vi "M227 Test Panel.vi"() -> ()   [LabVIEW 2020]
uses:
  <vilib>/Instr/_visa.llb/VISA Configure Serial Port (Instr).vi
panel:
  out "Waiting for Reply":bool
  out "Axis 3 Position":dbl
  out "Axis 2 Position":dbl
  out "Axis 1 Position":dbl
  in  "Move All (mm)":dbl
  out "Last Error":errorcluster
  out "Command History":string
  out "Reply":string
  in  "Command":string
  out "Connected":bool
  in  "Quit":bool
  in  "COM Port":refnum<visa-resource-name>="COM4"
  # "Example Commands:\n\nGet info for contoller 1\n1 *IDN?\n\nGet info for contoller 2\n2 *IDN?\n\nGet info for contoller 3\n3 *IDN?\n\nGet position of axis 1\n1 POS?\n\nGet position of axis 2\n2 POS?\n\nGet position of axis 2\n3 POS?\n\nMove axis 1 to a position of +1.5 mm\n1 MOV 1 1.5\n\nMove axis 2 to a position of +1.5 mm\n2 MOV 1 1.5\n\nMove axis 2 to a position of +1.5 mm\n3 MOV 1 1.5"
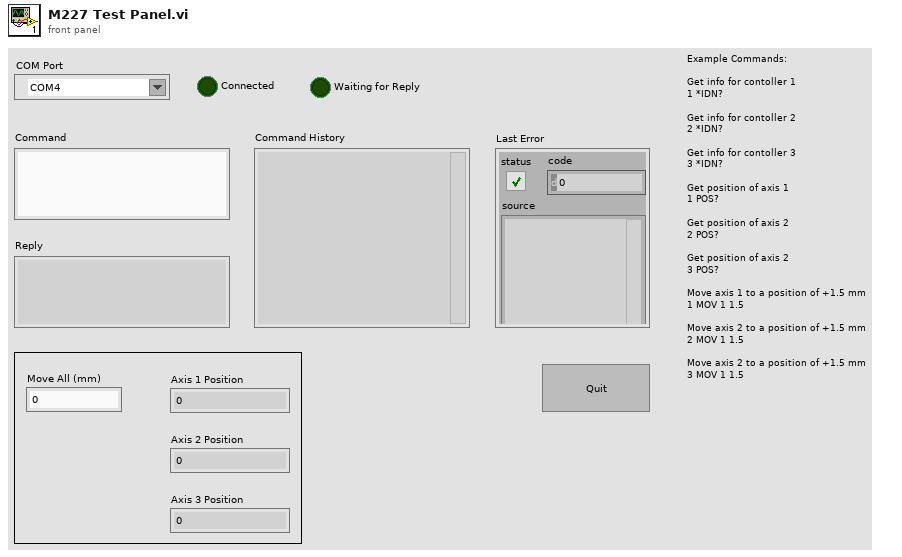
[diagram p1: front panel]
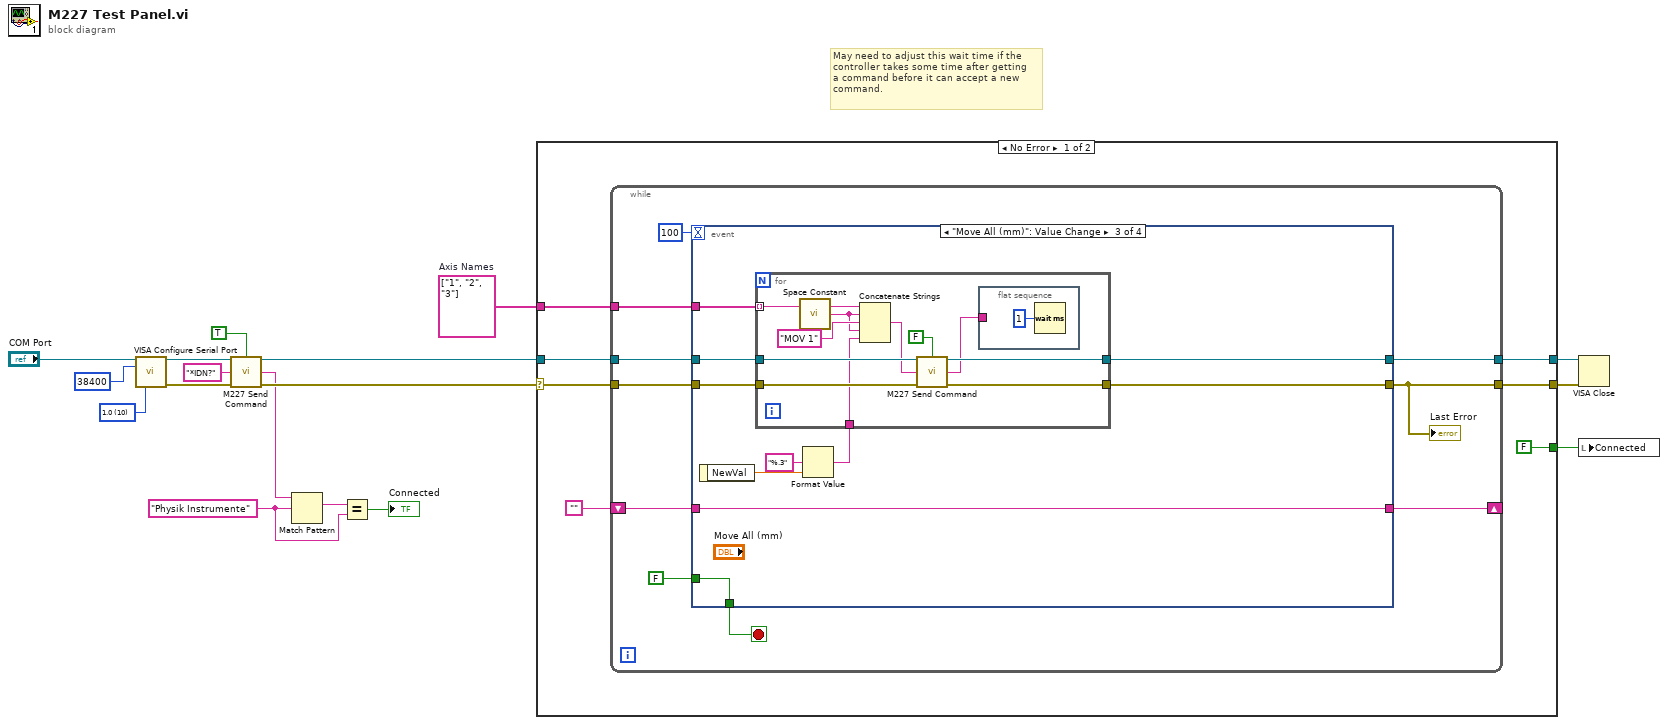
[diagram p0: block diagram]
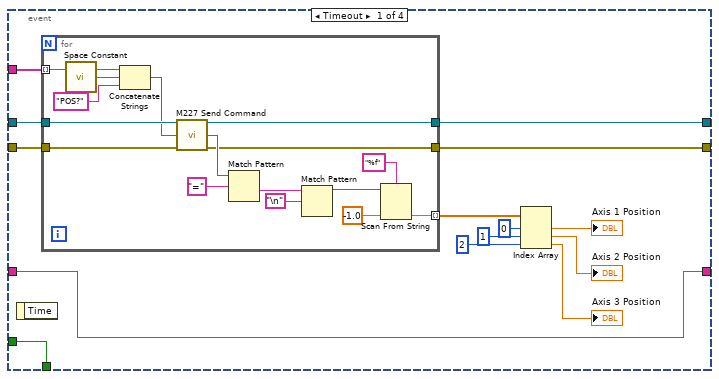
[diagram p2: hidden frame]
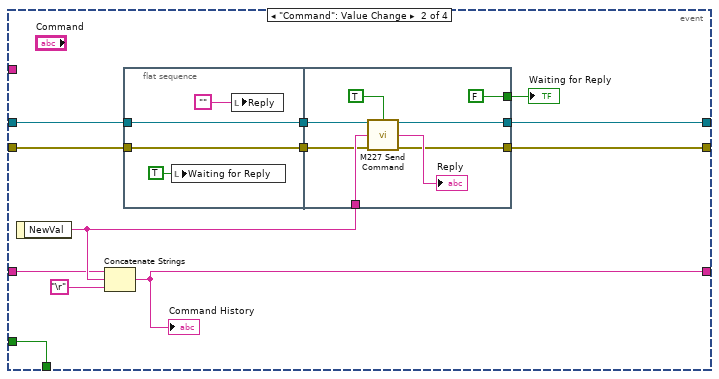
[diagram p3: hidden frame]
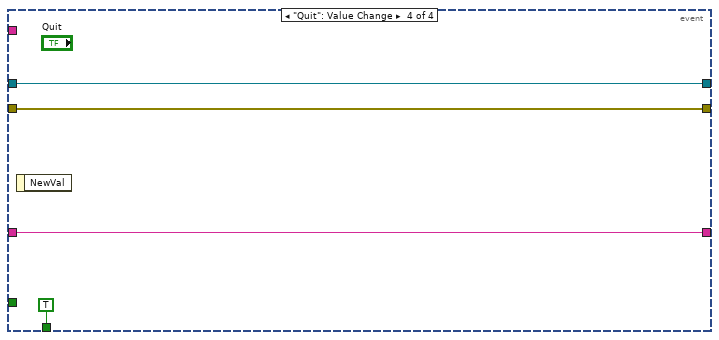
[diagram p4: hidden frame]
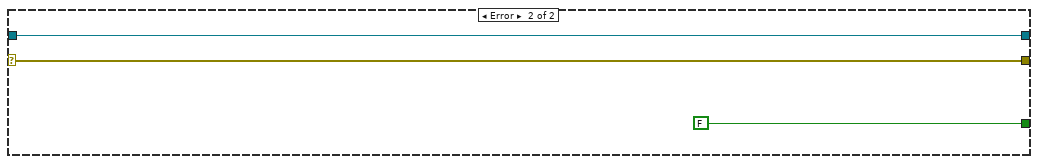
[diagram p5: hidden frame]
diagram:
  w1 = string[] ["1", "2", "3"]  # Axis Names
  w4 = "Physik Instrumente" ("regular expression")
  w17 = u16 10 items=["1.0"=10, "1.5"=15, "2.0"=20] ("stop bits (10: 1 bit)")
  # "May need to adjust this wait time if the\ncontroller takes some time after getting\na command before it can accept a new\ncommand."
  n1 = call-poly "VISA Configure Serial Port"("VISA resource name"="COM Port", "baud rate (9600)"=u32 38400, "stop bits (10: 1 bit)"=w17) -> ("VISA resource name out"=w12:refnum<visa-resource-name>, "error out"=w10:errorcluster)  [unwired: 11 in]
  n2 = call "M227 Send Command.vi"("VISA Ref"=w12, "Wait for Reply (T)"=TRUE, "Command"="*IDN?", "Error In"=w10) -> ("VISA Ref Dup"=w11:refnum<visa-resource-name>, "Reply"=w6:string, "Error Out"=w9:errorcluster)  [unwired: 9 in]
  n3 = Match Pattern(string=w6, regular expression=w4) -> (match substring=w5:string)  [unwired: 1 in, 3 out]
  n4 = Equal?(x=w5, y=w4) -> (x = y?=→"Connected":bool)
  n5 = case shown="No Error" w9 {
    selector: w9 -> [w23 w116]
    tunnel: w11 -> [w24 w117]
    tunnel: [w22 w117] -> w14
    tunnel: [w21 w116] -> w13
    tunnel: [FALSE FALSE] -> w2
    tunnel: w1 -> [w18 _]
    frame No Error {
      n6 = while {
        tunnel: w24 -> [w32]
        tunnel: w23 -> [w31]
        tunnel: [w30] -> w22
        tunnel: [w27] -> w21
        shift-right: [w28] -> _
        shift-left: "" -> [w29]
        tunnel: w18 -> [w25]
        stop <- w33 stop-if-true
        n7 = event shown="[2] \"Move All (mm)\": Value Change" {
          selector: _ -> [_ _ _ _]
          dyn-events: _ -> [_ _ _ _]
          timeout: 100 -> [_ _ _ _]
          tunnel: FALSE -> [w48 w76 w98 _]
          tunnel: [w48 w76 w98 TRUE] -> w33
          tunnel: w32 -> [w46 w75 w97 w114]
          tunnel: w31 -> [w45 w74 w96 w113]
          tunnel: [w44 w70 w91 w114] -> w30
          tunnel: [w43 w71 w90 w113] -> w27
          tunnel: w29 -> [w38 w67 w89 w111]
          tunnel: [w38 w66 w89 w111] -> w28
          tunnel: w25 -> [w47 _ w95 _]
          event Timeout {
            n8 = event-data() -> ()  [unwired: 1 in, 1 out]
            n9 = for {
              tunnel: w47 -> [w63] mode=indexing
              tunnel: w46 -> [w64]
              tunnel: w45 -> [w59]
              tunnel: [w51] -> w42 mode=indexing
              tunnel: [w50] -> w44
              tunnel: [w49] -> w43
              n10 = call <vilib>:"Space Constant.vi"() -> ("String"=w61:string)
              n11 = Concatenate Strings(w63, w61, "POS?") -> (w60:string)
              n12 = call "M227 Send Command.vi"("VISA Ref"=w64, "Command"=w60, "Error In"=w59) -> ("VISA Ref Dup"=w50:refnum<visa-resource-name>, "Reply"=w58:string, "Error Out"=w49:errorcluster)  [unwired: 10 in]
              n13 = Match Pattern(string=w58, regular expression="=") -> (after substring=w56:string)  [unwired: 1 in, 3 out]
              n14 = Match Pattern(string=w56, regular expression="\n") -> (before substring=w52:string)  [unwired: 1 in, 3 out]
              n15 = Scan From String(format string="%f", input string=w52, default 1=-1.0 ("default (0 dbl)")) -> (output 1=w51:dbl)  [unwired: 2 in, 3 out]
            }
            n16 = Index Array(array=w42, index #1=0 ("index"), index #2=1 ("index"), index #3=2 ("index")) -> (element #1=→"Axis 1 Position":dbl, element #2=→"Axis 2 Position":dbl, element #3=→"Axis 3 Position":dbl)
          }
          event "Command": Value Change {
            n17 = event-data() -> ("NewVal"=w69:string)  [unwired: 1 in]
            n18 = Concatenate Strings(w67, w69, "\r") -> (w66:string)
            "Command History" <- w66
            n19 = flat-sequence {
              tunnel: w74 -> [w79]
              tunnel: w75 -> [w80]
              tunnel: [w80] -> w73
              tunnel: [w79] -> w72
              tunnel: w69 -> [w86]
              tunnel: w73 -> [w88]
              tunnel: w72 -> [w85]
              tunnel: [w83] -> w71
              tunnel: [w82] -> w70
              tunnel: [FALSE] -> w65
              frame #0 {
                n20 = local write "Waiting for Reply"(TRUE ("Waiting for Cmd")) -> ()
                n21 = local write "Reply"("") -> ()
              }
              frame #1 {
                n22 = call "M227 Send Command.vi"("VISA Ref"=w88, "Wait for Reply (T)"=TRUE, "Command"=w86, "Error In"=w85) -> ("VISA Ref Dup"=w82:refnum<visa-resource-name>, "Reply"=→"Reply":string, "Error Out"=w83:errorcluster)  [unwired: 9 in]
              }
            }
            "Waiting for Reply" <- w65
          }
          event "Move All (mm)": Value Change {
            n23 = event-data() -> ("NewVal"=w94:dbl)  [unwired: 1 in]
            n24 = Format Value(format string="%.3", value (0)=w94) -> (output string=w92:string)  [unwired: 1 in]
            n25 = for {
              tunnel: w95 -> [w108] mode=indexing
              tunnel: w97 -> [w109]
              tunnel: w96 -> [w105]
              tunnel: [w104] -> w91
              tunnel: [w103] -> w90
              tunnel: w92 -> [w101]
              n26 = call <vilib>:"Space Constant.vi"() -> ("String"=w102:string)
              n27 = Concatenate Strings(w108, w102, "MOV 1", w102, w101) -> (w106:string)
              n28 = call "M227 Send Command.vi"("VISA Ref"=w109, "Wait for Reply (T)"=FALSE, "Command"=w106, "Error In"=w105) -> ("VISA Ref Dup"=w104:refnum<visa-resource-name>, "Reply"=w99:string, "Error Out"=w103:errorcluster)  [unwired: 9 in]
              n29 = flat-sequence {
                tunnel: w99 -> [_]
                frame #0 {
                  n30 = Wait (ms)(milliseconds to wait=u32 1) -> ()  [unwired: 1 out]
                }
              }
            }
          }
          event "Quit": Value Change {
            n31 = event-data() -> ()  [unwired: 1 in, 1 out]
          }
        }
        "Last Error" <- w27
      }
    }
    frame Error {
    }
  }
  n32 = VISA Close(VISA resource name=w14, error in (no error)=w13) -> ()  [unwired: 1 out]
  n33 = local write "Connected"(w2) -> ()
